vi "Memory (DBL).vi"(2 "initialize":bool, 3 "initial condition":dbl format="%.2f", 5 "input point":dbl format="%.2f") -> (1 "output point":dbl format="%.2f")   [LabVIEW 2017, in "NI_AdvCtrl_nonlinear.lvlib"]
doc: "LabVIEW no longer supports this VI. You can obtain similar functionality by installing the LabVIEW Simulation Module.\n\nStores the input value. It is output(n)=input(n-1), where output(0)=initial condition."
uses:
  <vilib>/addons/control/advanced/NI_AdvCtrl_nonlinear.lvlib
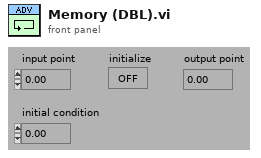
[diagram p1: front panel]
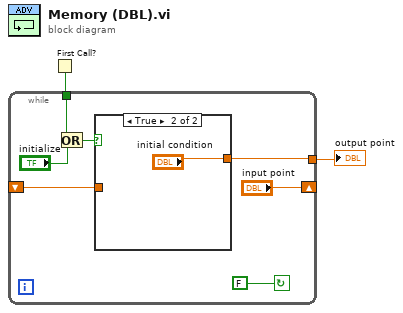
[diagram p0: block diagram]
diagram:
  n1 = First Call?() -> (First Call?: T/F=w1:bool)
  n2 = while {
    tunnel: w1 -> [w3]
    tunnel: [w8] -> w2
    shift-left: _ -> [w7]
    shift-right: ["input point"] -> _
    stop <- FALSE continue-if-true
    n3 = Or(x=w3, y="initialize") -> (x .or. y?=w5:bool)
    n4 = case shown="True" w5 {
      tunnel: [w10 "initial condition"] -> w8
      tunnel: w7 -> [w10 _]
      frame False {
      }
      frame True {
      }
    }
  }
  "output point" <- w2
